vi "Realy Output Post Sub Steps Batch.vi"(9 "Socket No":u16=1, 10 "RelayOutputWrite":T1, 11 "Sequence Context In":refnum<k7>) -> (0 "error out":errorcluster, 2 "PhysicalChannel":string[](array[string]), 3 "Report Text":string)   [LabVIEW 2023, in "LTT_TeststandSteptypes.lvlib"]
uses:
  LTT_TeststandSteptypes.lvlib
  Control/Relay Output.ctl
  <instrlib>/niSwitch/niSwitch.llb/niSwitch Topologies.ctl
  HardwareAbstractionLayer_LVOOP/NI Switch/NISwitch_class/NISwitch.lvclass
  <instrlib>/niSwitch/niSwitch.llb/niSwitch Relay Action.ctl
  HardwareAbstractionLayer_LVOOP/Digital Output/NI Digital Output_class/NI Digital Output.lvclass
  HardwareAbstractionLayer_LVOOP/Database/Database.lvclass
  HardwareAbstractionLayer_LVOOP/Database/SQL Public VI/Control/DB Options.ctl
panel:
  in  "error in":errorcluster
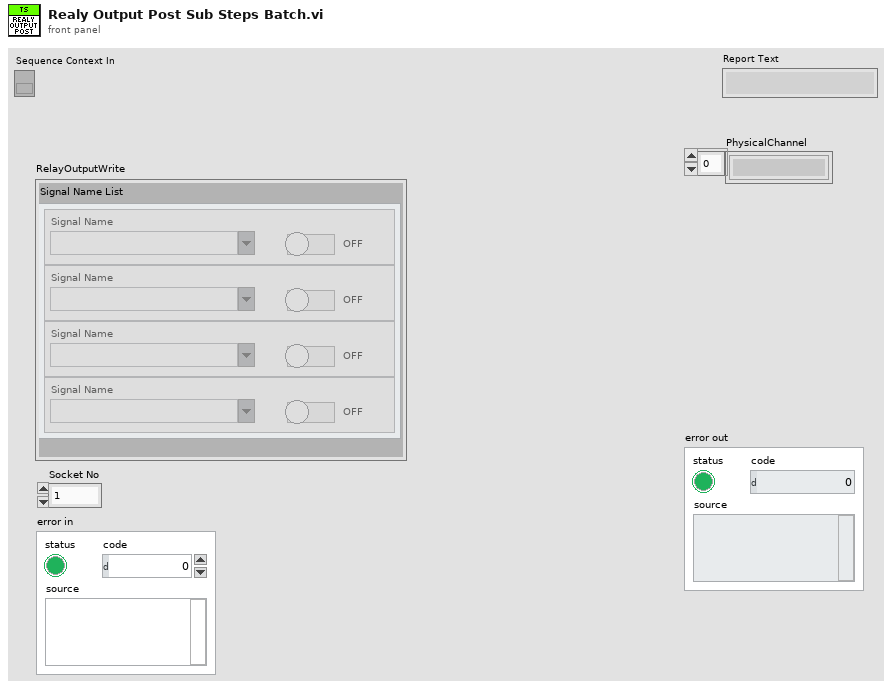
[diagram p1: front panel]
types:
  T1 = typedef "LTT_TeststandSteptypes.lvlib/Relay Output.ctl" = cluster{"Signal Name List":cluster{"Signal Name":string, "Enable Output":bool}[]}
  T2 = typedef "niSwitch Topologies.ctl" = string
  T3 = cluster{"Signal Name":string, "Enable Output":bool}[]
  T4 = typedef "HardwareAbstractionLayer_LVOOP.lvlib/Database.lvclass/DB Options.ctl" = enum16{"Init", "Select Data", "Insert Data", "Update Data", "Delete Data", "Execute Query", "Create Schema", "Create Table", "List Tables", "List Columns", "Close"}
  T5 = cluster{"table":string, "condition":string, "columns":string[]}
  T6 = typedef "niSwitch Relay Action.ctl" = i32
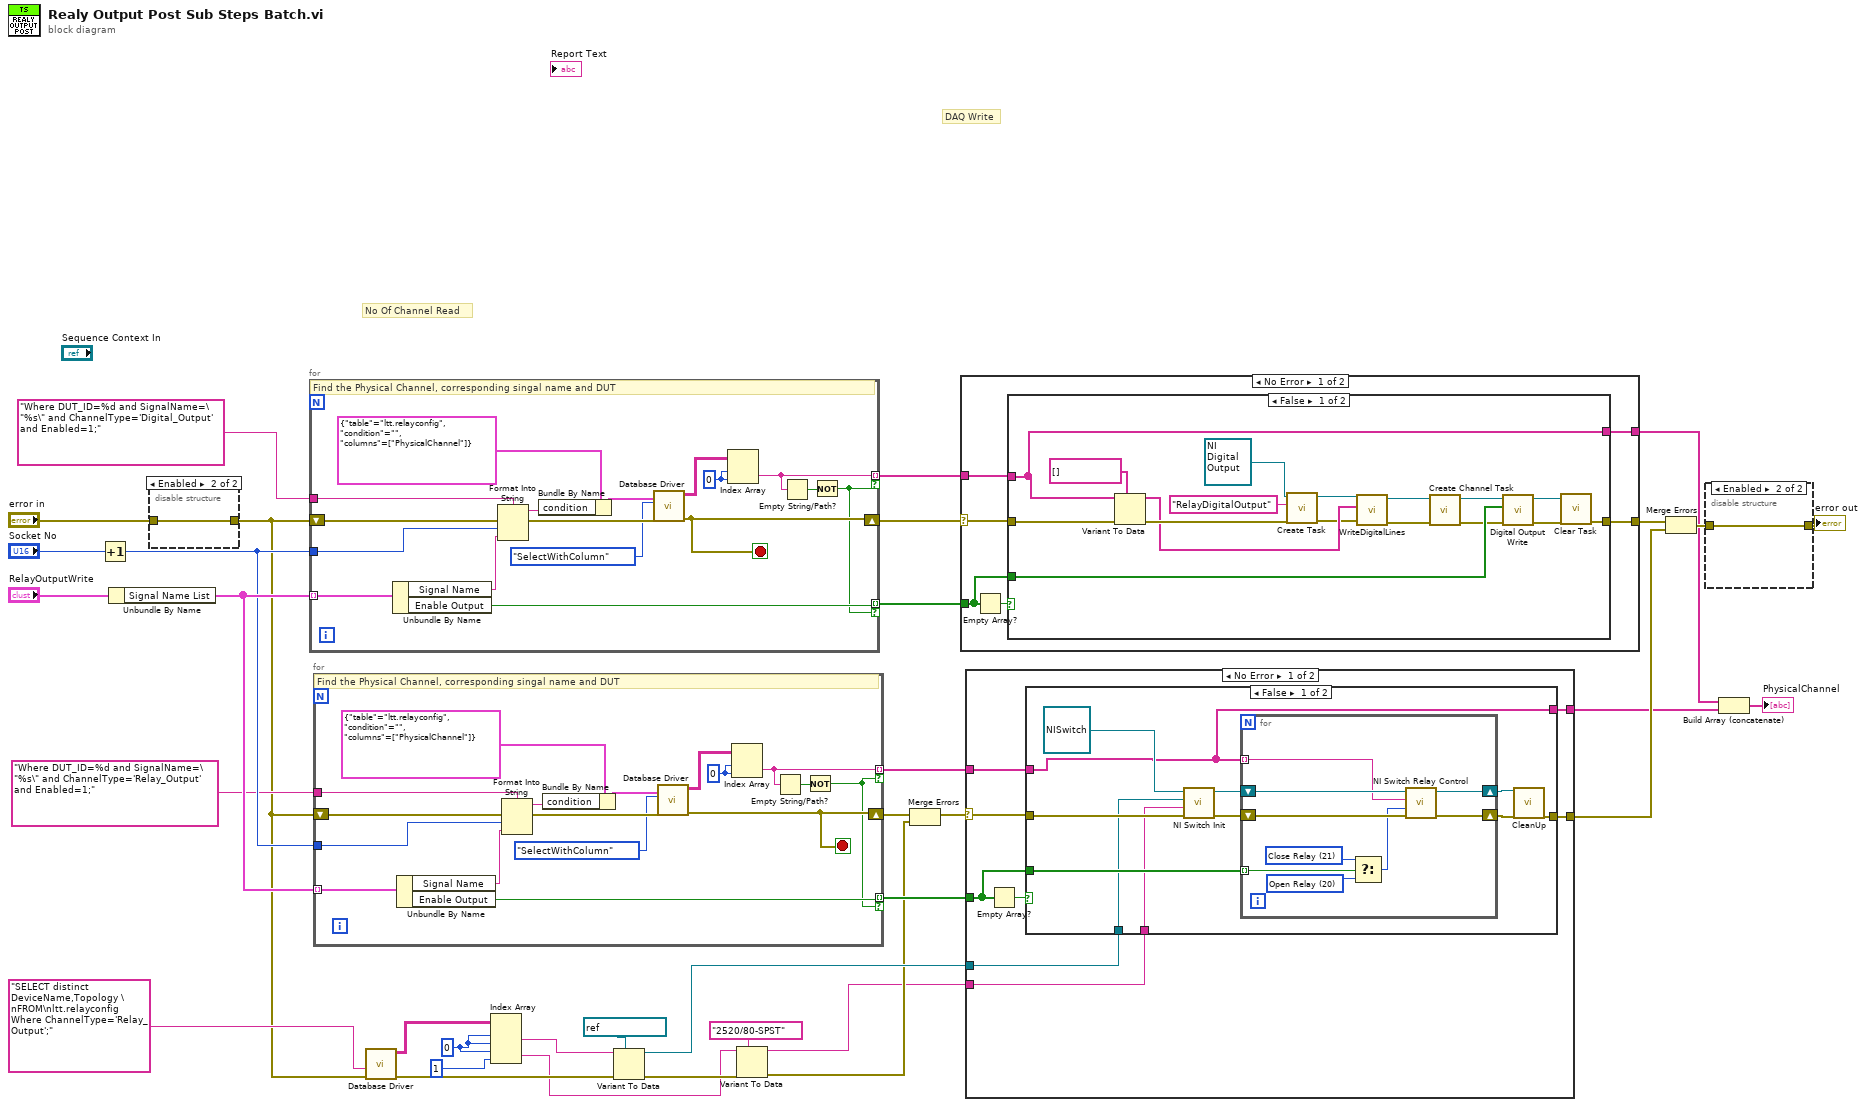
[diagram p0: block diagram]
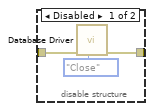
[diagram p2: hidden frame]
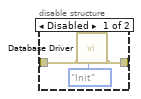
[diagram p3: hidden frame]
diagram:
  w13 = 0 ("disabled index (col)")
  # "DAQ Write"
  # "No Of Channel Read"
  n1 = Increment(x="Socket No") -> (x+1=w27:u16)
  n2 = Unbundle By Name("RelayOutputWrite") -> ("Signal Name List"=w28:T3)
  n3 = disable-structure shown="Enabled" {
    disable-tunnel: "error in" -> [w37 w39]
    disable-tunnel: [w36 w39] -> w6
    frame Disabled {
      n4 = call "Database Driver.vi"("Options"=DB_Options."Init", "error in"=w37) -> ("error out"=w36:errorcluster)  [unwired: 6 in, 3 out]
    }
    frame Enabled {
    }
  }
  n5 = for {
    tunnel: w28 -> [w46] mode=indexing
    tunnel: "Where DUT_ID=%d and SignalName=\"%s\" and ChannelType='Digital_Output' and Enabled=1;" -> [w56]
    shift-right: [w49] -> w31
    shift-left: w6 -> [w52]
    tunnel: w27 -> [w48]
    tunnel: [w44] -> w33 mode=indexing if=w40
    tunnel: [w42] -> w32 mode=indexing if=w40
    stop <- w49 stop-if-true
    w50 = 0 ("disabled index (col)")
    # "Find the Physical Channel, corresponding singal name and DUT"
    n6 = Unbundle By Name(w46) -> ("Signal Name"=w45:string, "Enable Output"=w44:bool)
    n7 = Format Into String(format string=w56, error in=w52, w48, w45) -> (resulting string=w54:string, error out=w51:errorcluster)  [unwired: 1 in]
    n8 = Bundle By Name(cluster=T5 {"table"="ltt.relayconfig", "condition"="", "columns"=["PhysicalChannel"]} ("SQLTableData"), "condition"=w54) -> (w53:T5)
    n9 = call "Database Driver.vi"("SQLTableData"=w53, "error in"=w51, "Select"=enum16{"SelectWithQuery", "SelectWithColumn"}."SelectWithColumn") -> ("error out"=w49:errorcluster, "data"=w43:string[][])  [unwired: 5 in, 2 out]
    n10 = Index Array(array=w43, index (row)=w50, index (col)=w50) -> (element=w42:string)
    n11 = Empty String/Path?(string/path=w42) -> (empty?=w41:bool)
    n12 = Not(x=w41) -> (.not. x?=w40:bool)
  }
  n13 = for {
    tunnel: w28 -> [w64] mode=indexing
    shift-right: [w67] -> w26
    shift-left: w6 -> [w70]
    tunnel: w27 -> [w66]
    tunnel: [w62] -> w25 mode=indexing if=w57
    tunnel: [w58] -> w22 mode=indexing if=w57
    tunnel: "Where DUT_ID=%d and SignalName=\"%s\" and ChannelType='Relay_Output' and Enabled=1;" -> [w60]
    stop <- w67 stop-if-true
    w68 = 0 ("disabled index (col)")
    # "Find the Physical Channel, corresponding singal name and DUT"
    n14 = Unbundle By Name(w64) -> ("Signal Name"=w63:string, "Enable Output"=w62:bool)
    n15 = Format Into String(format string=w60, error in=w70, w66, w63) -> (resulting string=w72:string, error out=w69:errorcluster)  [unwired: 1 in]
    n16 = Bundle By Name(cluster=T5 {"table"="ltt.relayconfig", "condition"="", "columns"=["PhysicalChannel"]} ("SQLTableData"), "condition"=w72) -> (w71:T5)
    n17 = call "Database Driver.vi"("SQLTableData"=w71, "error in"=w69, "Select"=enum16{"SelectWithQuery", "SelectWithColumn"}."SelectWithColumn") -> ("error out"=w67:errorcluster, "data"=w61:string[][])  [unwired: 5 in, 2 out]
    n18 = Index Array(array=w61, index (row)=w68, index (col)=w68) -> (element=w58:string)
    n19 = Empty String/Path?(string/path=w58) -> (empty?=w59:bool)
    n20 = Not(x=w59) -> (.not. x?=w57:bool)
  }
  n21 = call "Database Driver.vi"("error in"=w6, "SQL query"="SELECT distinct DeviceName,Topology \nFROM\nltt.relayconfig Where ChannelType='Relay_Output';") -> ("error out"=w19:errorcluster, "data"=w21:string[][])  [unwired: 6 in, 2 out]
  n22 = Index Array(array=w21, index (row) #1=w13, index (col) #1=w13, index (row) #2=w13, index (col) #2=1 ("disabled index (col)")) -> (element #1=w20:string, element #2=w17:string)
  n23 = Variant To Data(error in=w19, type=refnum<k15> "PXI2Slot17" ("resource name"), Variant=w20) -> (data=w11:refnum<k15>, error out=w18:errorcluster)
  n24 = Variant To Data(error in=w18, type=T2 "2520/80-SPST" ("topology name"), Variant=w17) -> (data=w8:T2, error out=w9:errorcluster)
  n25 = Merge Errors(w26, w9) -> (w10:errorcluster)
  n26 = case shown="No Error" w31 {
    selector: w31 -> [w77 w98]
    tunnel: w33 -> [w76 _]
    tunnel: w32 -> [w78 _]
    tunnel: [w75 w98] -> w29
    tunnel: [w74 _] -> w3
    frame No Error {
      n27 = Empty Array?(array=w76) -> (empty?=w79:bool)
      n28 = case shown="False" w79 {
        tunnel: w78 -> [w80 _]
        tunnel: w77 -> [w96 w97]
        tunnel: w76 -> [w88 _]
        tunnel: [w86 w97] -> w75
        tunnel: [w80 _] -> w74
        frame False {
          n29 = Variant To Data(error in=w96, type=tag[] [] ("DigitalLines"), Variant=w80) -> (data=w92:tag[], error out=w95:errorcluster)
          n30 = call-dynamic "Create Task.vi"("error in"=w95, "Task Name"="RelayDigitalOutput", "NI Digital Output in"=refnum<class "NI Digital Output.lvclass"> refnum ("HardwareAbstractionLayer_LVOOP.lvlib:NI Digital Output.lvclass")) -> ("error out"=w89:errorcluster, "NI Digital Output out"=w93:refnum<class "NI Digital Output.lvclass">)  [unwired: 7 in]
          n31 = call-dynamic "WriteDigitalLines.vi"("error in (no error)"=w89, "DigitalLines"=w92, "NI Digital Output in"=w93) -> ("error out"=w83:errorcluster, "NI Digital Output out"=w85:refnum<class "NI Digital Output.lvclass">)  [unwired: 7 in]
          n32 = call-dynamic "Create Channel Task.vi"("error in"=w83, "NI Digital Output in"=w85) -> ("error out"=w82:errorcluster, "NI Digital Output out"=w84:refnum<class "NI Digital Output.lvclass">)  [unwired: 8 in]
          n33 = call-dynamic "Digital Output Write.vi"("error in"=w82, "Digital Output Write"=w88, "NI Digital Output in"=w84) -> ("error out"=w81:errorcluster, "NI Digital Output out"=w87:refnum<class "NI Digital Output.lvclass">)  [unwired: 7 in]
          n34 = call-dynamic "Clear Task.vi"("error in"=w81, "NI Digital Output in"=w87) -> ("error out"=w86:errorcluster)  [unwired: 8 in, 1 out]
        }
        frame True {
        }
      }
    }
    frame Error {
    }
  }
  n35 = case shown="No Error" w10 {
    selector: w10 -> [w102 w128]
    tunnel: w25 -> [w105 _]
    tunnel: [w104 w128] -> w24
    tunnel: w22 -> [w103 _]
    tunnel: w11 -> [w101 _]
    tunnel: w8 -> [w100 _]
    tunnel: [w99 _] -> w2
    frame No Error {
      n36 = Empty Array?(array=w105) -> (empty?=w106:bool)
      n37 = case shown="False" w106 {
        tunnel: w102 -> [w116 w127]
        tunnel: w105 -> [w110 _]
        tunnel: [w111 w127] -> w104
        tunnel: w103 -> [w107 _]
        tunnel: w101 -> [w109 _]
        tunnel: w100 -> [w108 _]
        tunnel: [w107 _] -> w99
        frame False {
          n38 = call "NI Switch Init.vi"("error in (no error)"=w116, "topology name"=w108, "resource name"=w109, "object in"=refnum<class "NISwitch.lvclass"> refnum ("HardwareAbstractionLayer_LVOOP.lvlib:RelayOutput")) -> ("error out"=w114:errorcluster, "object out"=w115:refnum<class "NISwitch.lvclass">)  [unwired: 6 in]
          n39 = for {
            shift-right: [w124] -> w113
            shift-left: w115 -> [w126]
            shift-right: [w123] -> w112
            shift-left: w114 -> [w125]
            tunnel: w110 -> [w121] mode=indexing
            tunnel: w107 -> [w118] mode=indexing
            w120 = T6 20 items=["Open Relay"=20, "Close Relay"=21] ("f")
            w122 = T6 21 items=["Open Relay"=20, "Close Relay"=21] ("relay action (Close Relay)")
            n40 = Select(t=w122, s=w121, f=w120) -> (s? t:f=w119:T6)
            n41 = call-dynamic "NI Switch Relay Control.vi"("error in (no error)"=w125, "relay action (Close Relay)"=w119, "relay names"=w118, "RelayOutput in"=w126) -> ("error out"=w123:errorcluster, "RelayOutput out"=w124:refnum<class "NISwitch.lvclass">)  [unwired: 6 in]
          }
          n42 = call-dynamic "CleanUp.vi"("object in"=w113, "error in (no error)"=w112) -> ("error out"=w111:errorcluster)  [unwired: 16 in, 1 out]
        }
        frame True {
        }
      }
    }
    frame Error {
    }
  }
  n43 = Merge Errors(w29, w24) -> (w5:errorcluster)
  n44 = disable-structure shown="Enabled" {
    disable-tunnel: w5 -> [w131 w132]
    disable-tunnel: [w130 w132] -> w4
    frame Disabled {
      n45 = call "Database Driver.vi"("Options"=DB_Options."Close", "error in"=w131) -> ("error out"=w130:errorcluster)  [unwired: 6 in, 3 out]
    }
    frame Enabled {
    }
  }
  "error out" <- w4
  n46 = Build Array (concatenate)(w3, w2) -> (→"PhysicalChannel":string[])
